vi "FinalizeListGeneration.vi"(8 "error in (no error)":errorcluster, 11 "CDependencyList in":refnum<class "CDependencyList.lvclass">) -> (0 "error out":errorcluster, 3 "CDependencyList out":refnum<class "CDependencyList.lvclass">)   [LabVIEW 2020, in "DependencyInspection.lvlib" / "CDependencyList.lvclass"]
uses:
  CDependencyList.lvclass
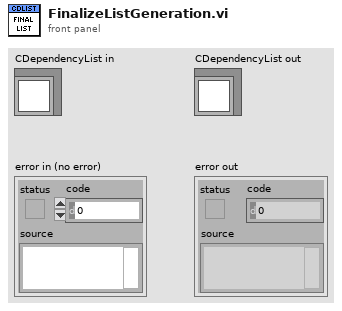
[diagram p1: front panel]
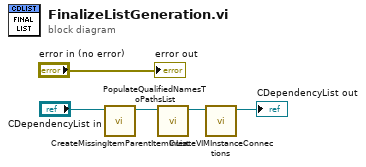
[diagram p0: block diagram]
diagram:
  n1 = call-dynamic "PopulateQualifiedNamesToPathsList.vi"("CDependencyList in"="CDependencyList in") -> ("CDependencyList out"=w4:refnum<class "CDependencyList.lvclass">)  [unwired: 9 in, 1 out]
  n2 = call-dynamic "CreateMissingItemParentItemInList.vi"("CDependencyList in"=w4) -> ("CDependencyList out"=w3:refnum<class "CDependencyList.lvclass">)  [unwired: 9 in, 1 out]
  n3 = call-dynamic "CreateVIMInstanceConnections.vi"("CDependencyList in"=w3) -> ("CDependencyList out"=→"CDependencyList out":refnum<class "CDependencyList.lvclass">)  [unwired: 9 in, 1 out]
  "error out" <- "error in (no error)"
